vi "SM Practice 2.vi"() -> ()   [LabVIEW 2020]
panel:
  out "x*y":dbl
  in  "stop":bool
  in  "Acquire":bool
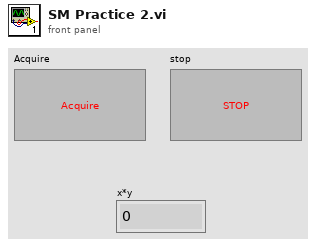
[diagram p1: front panel]
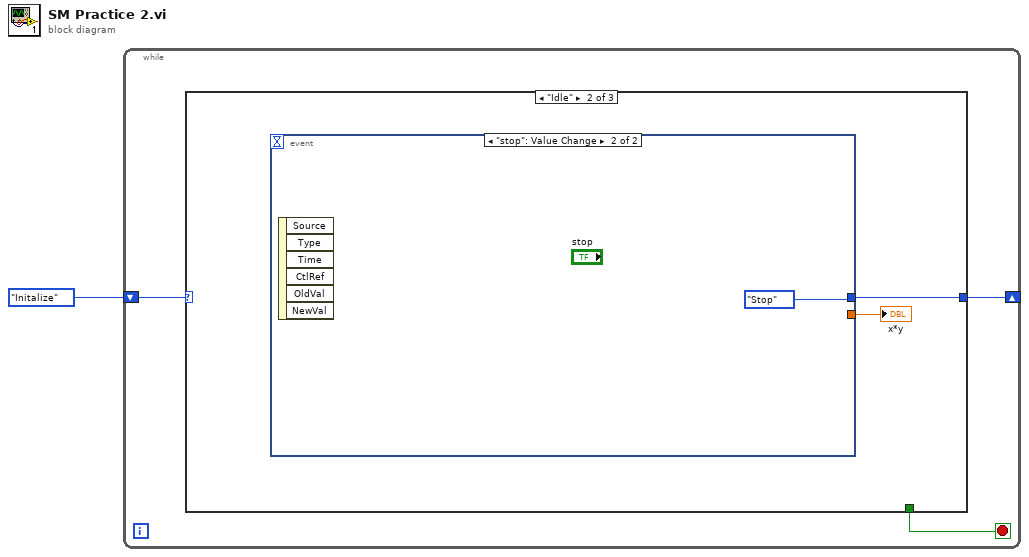
[diagram p0: block diagram]
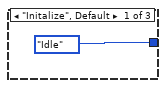
[diagram p2: hidden frame]
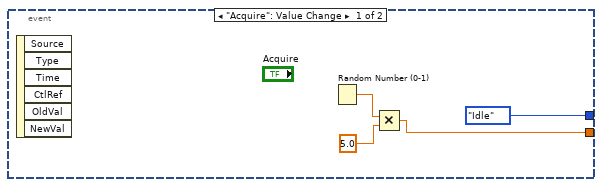
[diagram p3: hidden frame]
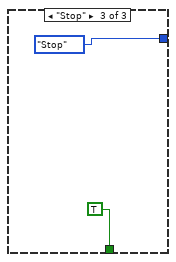
[diagram p4: hidden frame]
diagram:
  n1 = while {
    shift-right: [w2] -> _
    shift-left: enum16{"Initalize", "Idle", "Stop"}."Initalize" -> [w4]
    stop <- w3 stop-if-true
    n2 = case shown="\"Idle\"" w4 {
      tunnel: [enum16{"Initalize", "Idle", "Stop"}."Idle" w7 enum16{"Initalize", "Idle", "Stop"}."Stop"] -> w2
      tunnel: [_ _ TRUE] -> w3
      frame "Initalize", Default {
      }
      frame "Idle" {
        n3 = event shown="[1] \"stop\": Value Change" {
          selector: _ -> [_ _]
          dyn-events: _ -> [_ _]
          timeout: _ -> [_ _]
          tunnel: [enum16{"Initalize", "Idle", "Stop"}."Idle" enum16{"Initalize", "Idle", "Stop"}."Stop"] -> w7
          tunnel: [w8 _] -> w6
          event "Acquire": Value Change {
            n4 = event-data() -> ()  [unwired: 1 in, 6 out]
            n5 = Random Number (0-1)() -> (number: 0 to 1=w11:dbl)
            n6 = Multiply(x=w11, y=5.0) -> (x*y=w8:dbl)
          }
          event "stop": Value Change {
            n7 = event-data() -> ()  [unwired: 1 in, 6 out]
          }
        }
        "x*y" <- w6
      }
      frame "Stop" {
      }
    }
  }
